vi "Read Wrapper for BP Measurements.vi"(4 "Last Read":bool=TRUE, 6 "Timeout (ms)":i32, 7 "Data Element":T4, 8 "error in (no error)":errorcluster, 9 "Read Configuration":T2={"Read Position"=enum."Newest", "Element Offset"=0, "Prepend Array Size"=TRUE, "Get Read Position"=FALSE}, 10 "Data in":dbl[](array[numeric]), 11 "CIF_CIPC_Fifo_U8 in":refnum<class "CIF_CIPC_Fifo_DAQ.lvclass">) -> (0 "error out":errorcluster, 1 "Read Result Details":T1, 2 "Data out":dbl[](array[numeric]), 3 "CIF_CIPC_Fifo_U8 out":refnum<class "CIF_CIPC_Fifo_DAQ.lvclass">, 5 "Success":bool)   [LabVIEW 2021, in "CIF_CIPC_Fifo_DAQ.lvclass"]
uses:
  CIF_CIPC_Fifo_DAQ.lvclass
  D:/dev/Packages/CIF_Channels_Core/src/CIFChannels/CIFChannels.lvclass
  D:/dev/Packages/CIF_Channels_Core/src/CIPC_Channels/CIF_CIPC_Chan/CIF_CIPC_Chn.lvclass
  <vilib>/CIF Foundation/CIF CIPC/TypeDefs/Data Element Details.ctl
  <vilib>/CIF Foundation/CIF CIPC/TypeDefs/Read Configuration.ctl
  <vilib>/CIF Foundation/CIF CIPC/TypeDefs/Read Position.ctl
  <vilib>/CIF Foundation/CIF CIPC/TypeDefs/Read Result Details.ctl
  CIFChannels/CIFChannels.lvclass/CIFChannels.ctl
  CIF_CIPC_Chan/CIF_CIPC_Chn.lvclass/CIF_CIPC_Chn.ctl
  b5615cf0-cd7f-4476-b9a9-d6ef7628cc3b.vi
  6248fc70-cc83-4025-b778-a3221b95feac.vi
  CIFChannels/Accessors/Read FIFO Backpressure.vi
  <vilib>/CIF Foundation/CIF CIPC/SubVIs/Wait For N Elements Available.vi
  <vilib>/CIF Foundation/CIF CIPC/SubVIs/Get Element Read Position.vi
  <vilib>/CIF Foundation/CIF CIPC/SubVIs/Check Error.vi
  <vilib>/CIF Foundation/CIF CIPC/SubVIs/Get dll Path.vi
  <vilib>/CIF Foundation/CIF CIPC/SubVIs/Set Element Read Position.vi
  6248fc70-cc83-4025-b778-a3221b95feac.vi/331f6ecb-7ec4-4931-b93d-4fbd8d66a851.vi
  6248fc70-cc83-4025-b778-a3221b95feac.vi/5ce0d4cf-f921-42ba-b14c-c90f7f7611e4.vi
  <vilib>/CIF Foundation/CIF CIPC/SubVIs/Notify Of New Write.vi
  <vilib>/CIF Foundation/CIF CIPC/SubVIs/Get Element Write Position.vi
  <vilib>/Utility/error.llb/Trim Whitespace.vi
  <vilib>/Utility/error.llb/Error Cluster From Error Code.vi
  <vilib>/CIF Foundation/CIF CIPC/SubVIs/Get Element Info Variant.vi
  CIF_CIPC_Fifo_DAQ.lvclass/CIF_CIPC_Fifo_DAQ.ctl
  CIF_CIPC_Chan/CIF_CIPC_Chn.lvclass
  <vilib>/CIF Foundation/CIF CIPC/CIF_NI_CIPC.lvlib
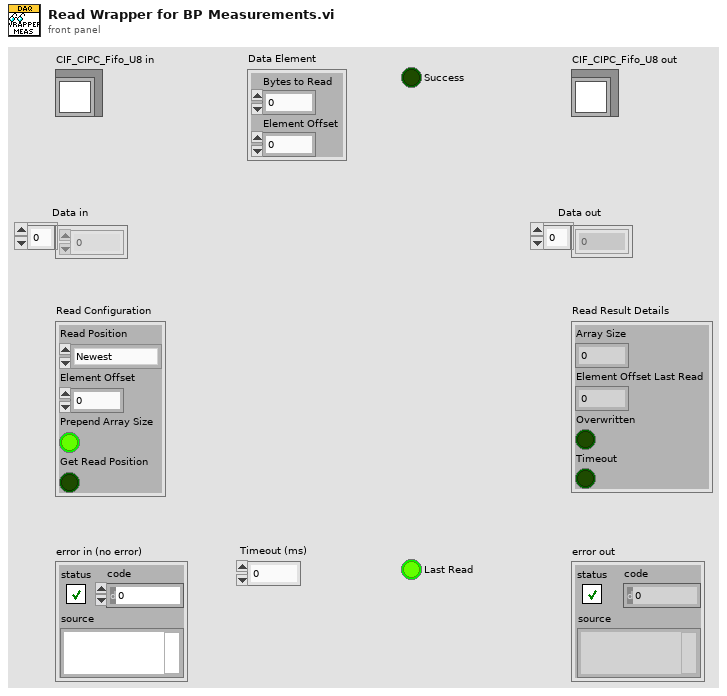
[diagram p1: front panel]
types:
  T1 = typedef "CIF_NI_CIPC.lvlib/Read Result Details.ctl" = cluster{"Array Size":i32, "Element Offset Last Read":u32, "Overwritten":bool, "Timeout":bool}
  T2 = typedef "CIF_NI_CIPC.lvlib/Read Configuration.ctl" = cluster{"Read Position":T3, "Element Offset":i32, "Prepend Array Size":bool, "Get Read Position":bool}
  T3 = typedef "CIF_NI_CIPC.lvlib/Read Position.ctl" = enum16{"Next", "Newest", "Oldest", "Next Available", "Absolute"}
  T4 = typedef "CIF_NI_CIPC.lvlib/Data Element Details.ctl" = cluster{"Bytes to Read":u32, "Element Offset":u32}
  T5 = typedef "CIF_CIPC_Chn.lvclass/Buffer Configuration Data.ctl" = cluster{"Total Size":u32, "Read Size":u32, "Read Offset":u32, "CIPC BP References":T6, "Override CIPC Name":string, "Encoder Data":string}
  T6 = typedef "CIF_NI_CIPC.lvlib/Backpressure References.ctl" = cluster{"CIPC Reference":u64, "CIPC BP Reference":u64}
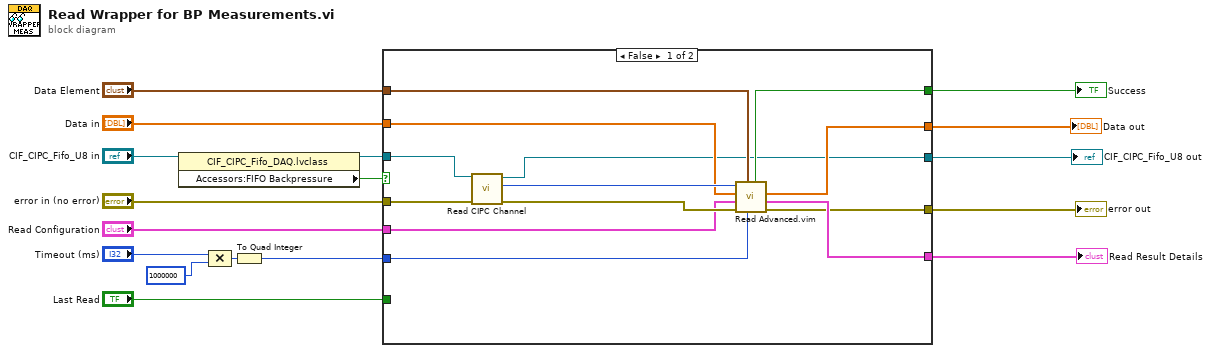
[diagram p0: block diagram]
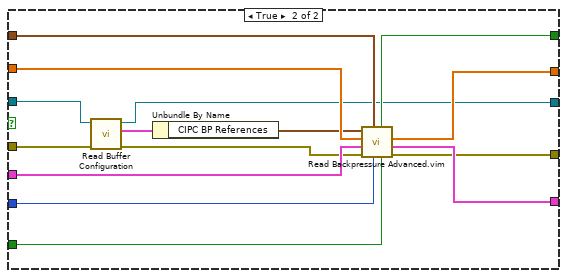
[diagram p2: hidden frame]
diagram:
  n1 = property class="CIF_CIPC_Fifo_DAQ.lvclass"(reference="CIF_CIPC_Fifo_U8 in") -> (reference out=w16:refnum<class "CIF_CIPC_Fifo_DAQ.lvclass">, "Accessors:FIFO Backpressure"=w17:bool)  [unwired: 1 in, 1 out]
  n2 = Compound Arithmetic op=MULTIPLY("Timeout (ms)", 1000000 ("value")) -> (w14:i32)
  n3 = To Quad Integer(1:w14) -> (0:w15:i64)
  n4 = case shown="False" w17 {
    tunnel: "Data Element" -> [w28 w45]
    tunnel: "Data in" -> [w27 w44]
    tunnel: "Read Configuration" -> [w26 w43]
    tunnel: [w25 w42] -> w2
    tunnel: [w24 w41] -> w6
    tunnel: [w23 w40] -> w4
    tunnel: [w22 w39] -> w3
    tunnel: "error in (no error)" -> [w21 w36]
    tunnel: w15 -> [w20 w38]
    tunnel: w16 -> [w19 w37]
    tunnel: [w18 w34] -> w5
    tunnel: "Last Read" -> [_ w31]
    frame False {
      n5 = call "Read CIPC Channel.vi"("error in (no error)"=w21, "CIFTag in"=w19) -> ("error out"=w29:errorcluster, "CIPC Channel"=w30:u64, "CIFTag out"=w18:refnum<class "CIF_CIPC_Fifo_DAQ.lvclass">)  [unwired: 7 in]
      n6 = call "Read Advanced.vim"("Timeout (ns)"=w20, "Data Element"=w28, "error in (no error)"=w29, "Read Configuration"=w26, "Data in"=w27, "CIPC Reference in"=w30) -> ("error out"=w22:errorcluster, "Read Result Details"=w23:T1, "Data out"=w24:dbl[], "Success"=w25:bool)  [unwired: 1 in, 1 out]
    }
    frame True {
      n7 = call "Read Buffer Configuration.vi"("error in (no error)"=w36, "CIF_CIPC_Chn in"=w37) -> ("error out"=w35:errorcluster, "Buffer Configuration"=w33:T5, "CIF_CIPC_Chn out"=w34:refnum<class "CIF_CIPC_Fifo_DAQ.lvclass">)  [unwired: 7 in]
      n8 = Unbundle By Name(w33) -> ("CIPC BP References"=w32:T6)
      n9 = call "Read Backpressure Advanced.vim"("Last Read"=w31, "Timeout (ns)"=w38, "Data Element"=w45, "error in (no error)"=w35, "Read Configuration"=w43, "Data in"=w44, "CIPC BP References in"=w32) -> ("error out"=w39:errorcluster, "Read Result Details"=w40:T1, "Data out"=w41:dbl[], "Success"=w42:bool)  [unwired: 1 out]
    }
  }
  "error out" <- w3
  "CIF_CIPC_Fifo_U8 out" <- w5
  "Success" <- w2
  "Data out" <- w6
  "Read Result Details" <- w4
